vi "Test.vi"() -> ()   [LabVIEW 2016, in "Path Track.lvlib"]
uses:
  Path Track.lvlib
  FGV Control.ctl
panel:
  out "Waveform Chart":cluster{"Angle":dbl, "Gyro":dbl}(graph)
  in  "Get ms ago":u32
  out "Gyro":dbl
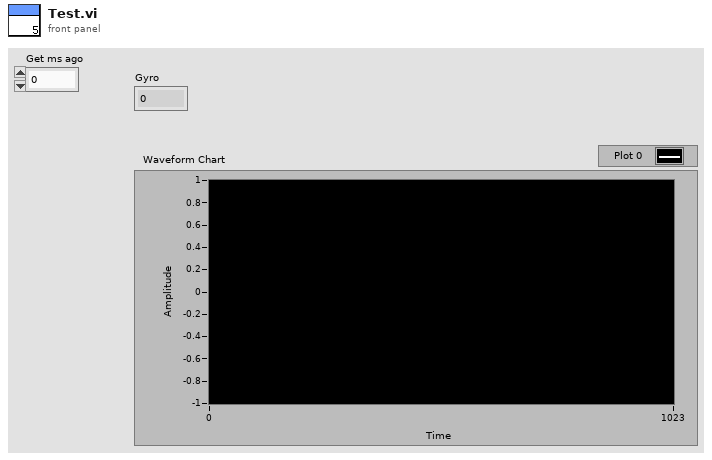
[diagram p1: front panel]
types:
  T1 = typedef "Path Track.lvlib/FGV Control.ctl" = enum16{"Allocate", "Get", "Append"}
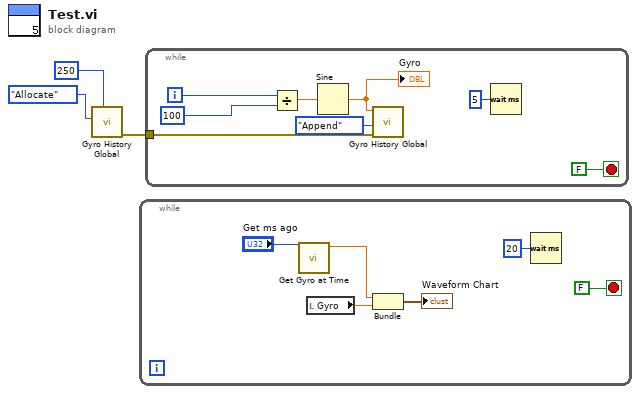
[diagram p0: block diagram]
diagram:
  n1 = call "Gyro History Global.vi"("Allocate Size"=250, "Operation"=FGV_Control."Allocate") -> ("error out"=w3:errorcluster)  [unwired: 8 in, 1 out]
  n2 = while {
    stop <- FALSE stop-if-true
    n3 = call "Get Gyro at Time.vi"("Get ms ago"="Get ms ago") -> ("Angle"=w5:dbl)  [unwired: 9 in, 1 out]
    n4 = local read "Gyro"() -> (w6:dbl)
    n5 = Bundle("Angle"=w5, "Gyro"=w6) -> (→"Waveform Chart":cluster{"Angle":dbl, "Gyro":dbl})  [unwired: 1 in]
    n6 = Wait (ms)(milliseconds to wait=u32 20) -> ()  [unwired: 1 out]
  }
  n7 = while {
    tunnel: w3 -> [w16]
    i -> [w15]
    stop <- FALSE stop-if-true
    n8 = Divide(x=w15, y=100) -> (x/y=w14:dbl)
    n9 = Sine(x=w14) -> (sin(x)=w12:dbl)
    "Gyro" <- w12
    n10 = call "Gyro History Global.vi"("error in"=w16, "Operation"=FGV_Control."Append", "Gyro"=w12) -> ()  [unwired: 7 in, 2 out]
    n11 = Wait (ms)(milliseconds to wait=u32 5) -> ()  [unwired: 1 out]
  }
